vi "Launcher Models.vi"(8 "error in (no error)":errorcluster, 11 "Controller in":refnum<class "Controller.lvclass">) -> (0 "error out":errorcluster, 3 "Controller out":refnum<class "Controller.lvclass">)   [LabVIEW 2020, in "Controller.lvlib" / "Controller.lvclass"]
uses:
  Controller.lvclass
  Models/Data Loader/Data Loader/Data Loader/Data Loader.lvclass
  C:/Program Files (x86)/National Instruments/LabVIEW 2020/vi.lib/ActorFramework/Actor/Actor.lvclass
  Models/Data Types/TDMS/TDMS.lvclass
  Models/Data Loader/Data Loader/Data Loader/Data Loader.lvclass/Data Loader.ctl
  Models/Data Loader/Data Loader/Data Loader/Accessor/Write Data File.lvclass.vi
  Depden On/MVVM Framework/MVVM Abstruct Controller/MVVM Abstruct Controller/MVVM Abstruct Controller.lvclass
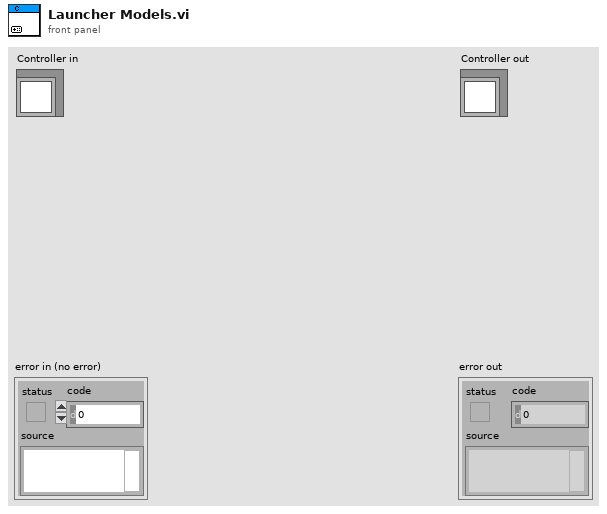
[diagram p1: front panel]
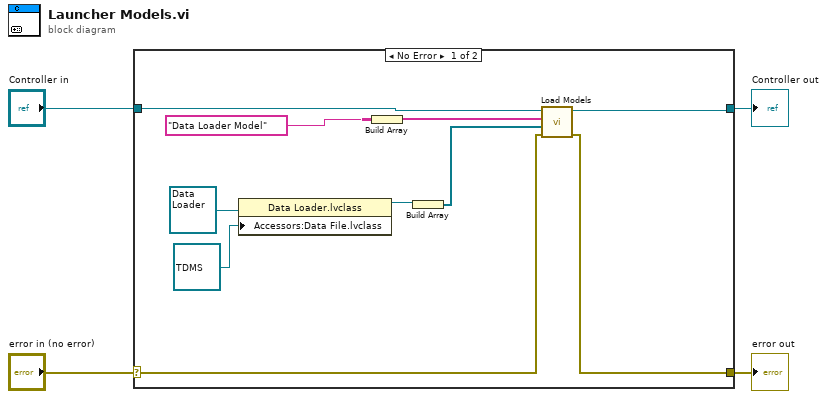
[diagram p0: block diagram]
diagram:
  n1 = case shown="No Error" "error in (no error)" {
    selector: "error in (no error)" -> [w6 w16]
    tunnel: [w5 w16] -> w3
    tunnel: [w13 w15] -> w1
    tunnel: "Controller in" -> [w14 w15]
    frame No Error {
      n2 = property class="Data Loader.lvclass"(reference=refnum<class "Data Loader.lvclass"> refnum ("Data Loader.lvlib:Data Loader.lvclass"), "Accessors:Data File.lvclass"=refnum<class "TDMS.lvclass"> refnum ("TDMS.lvclass")) -> (reference out=w8:refnum<class "Data Loader.lvclass">)  [unwired: 1 in, 1 out]
      n3 = Build Array("Data Loader Model") -> (w12:string[])
      n4 = Build Array(w8) -> (w7:refnum<class "Data Loader.lvclass">[])
      n5 = call "Load Models.vi"("error in (no error)"=w6, "Models"=w7, "Names"=w12, "MVVM Abstruct Controller in"=w14) -> ("error out"=w5:errorcluster, "MVVM Abstruct Controller out"=w13:refnum<class "Controller.lvclass">)  [unwired: 6 in]
    }
    frame Error {
    }
  }
  "error out" <- w3
  "Controller out" <- w1
